vi "SemiGreedy_Filters_(Top_Level_VI)-5.vi"(5 "[IN] Max angle":dbl, 6 "[IN] Dot matrix with statuses \nfor potentially moving dots":i16[][](array[numeric]), 7 "[IN] Possibly\nMoving (X,Y)":dbl[][](array[numeric]), 8 "error IN":errorcluster, 9 "[IN] Areas particles\nPrimary Detected":dbl[][](array[numeric]), 10 "[IN] Primary \n(X,Y) Detected":dbl[][](array[numeric]), 11 "[IN] Grouped tracks":T1(array[cluster])) -> (0 "error OUT":errorcluster, 2 "[OUT] Processed Tracks":T1(array[cluster]), 3 "[OUT Tracks before Processing":T1(array[cluster]))   [LabVIEW 2013]
panel:
  out "# Iteration":i32
  out "Current\ngroup":i32
  out "# of corrections":i32
  out "[IN] Before Pro\ncessing Tracks":T1(array[cluster])
  out "[IN] Current Pro\ncessing Tracks":T2
  out "[OUT] Clusters for Re\nconstructed Tracks":T2
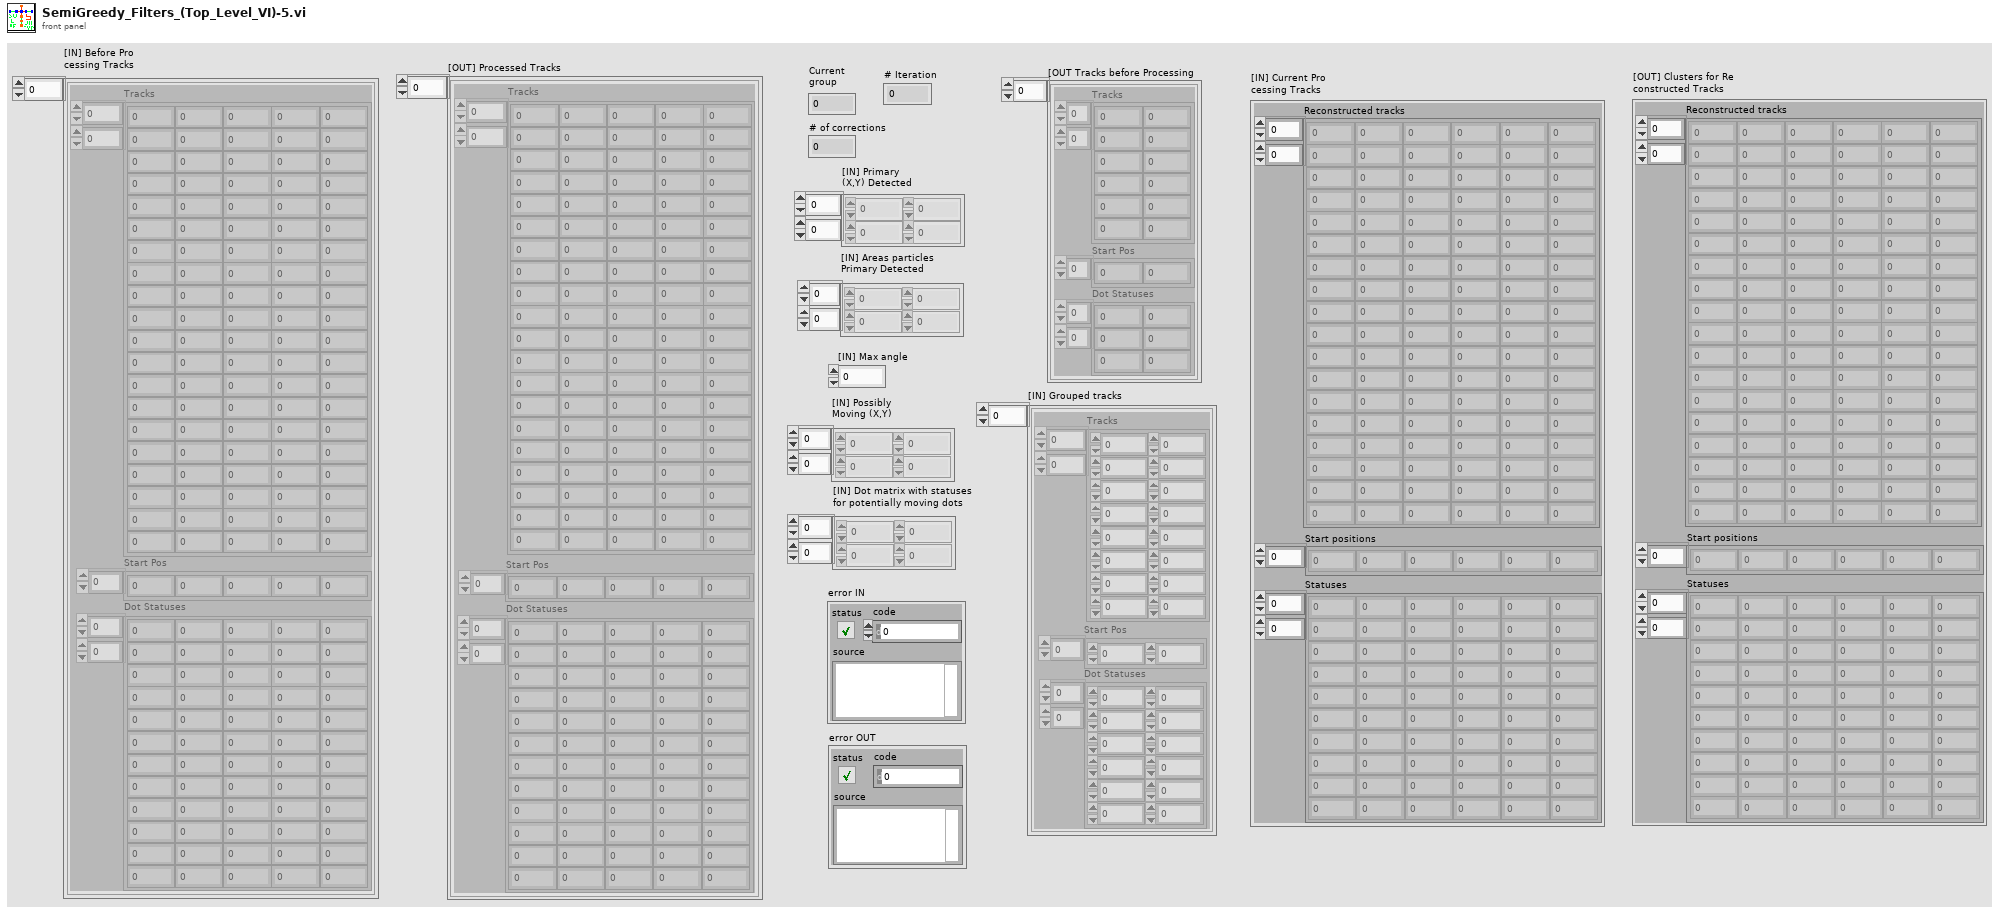
[diagram p1: front panel]
types:
  T1 = cluster{"Tracks":dbl[][], "Start Pos":i32[], "Dot Statuses":i16[][]}[]
  T2 = cluster{"Reconstructed tracks":dbl[][], "Start positions":i32[], "Statuses":i16[][]}
  T3 = cluster{"Tracks":dbl[][], "Start Pos":i32[], "Dot Statuses":i16[][]}
  T4 = cluster{"Subtrack":dbl[], "Statuses":i16[], "Start pos":i32, "Additions to cost":i32, "Track variant \nis too short":bool, "Indexes for Jumps":i32[]}[][]
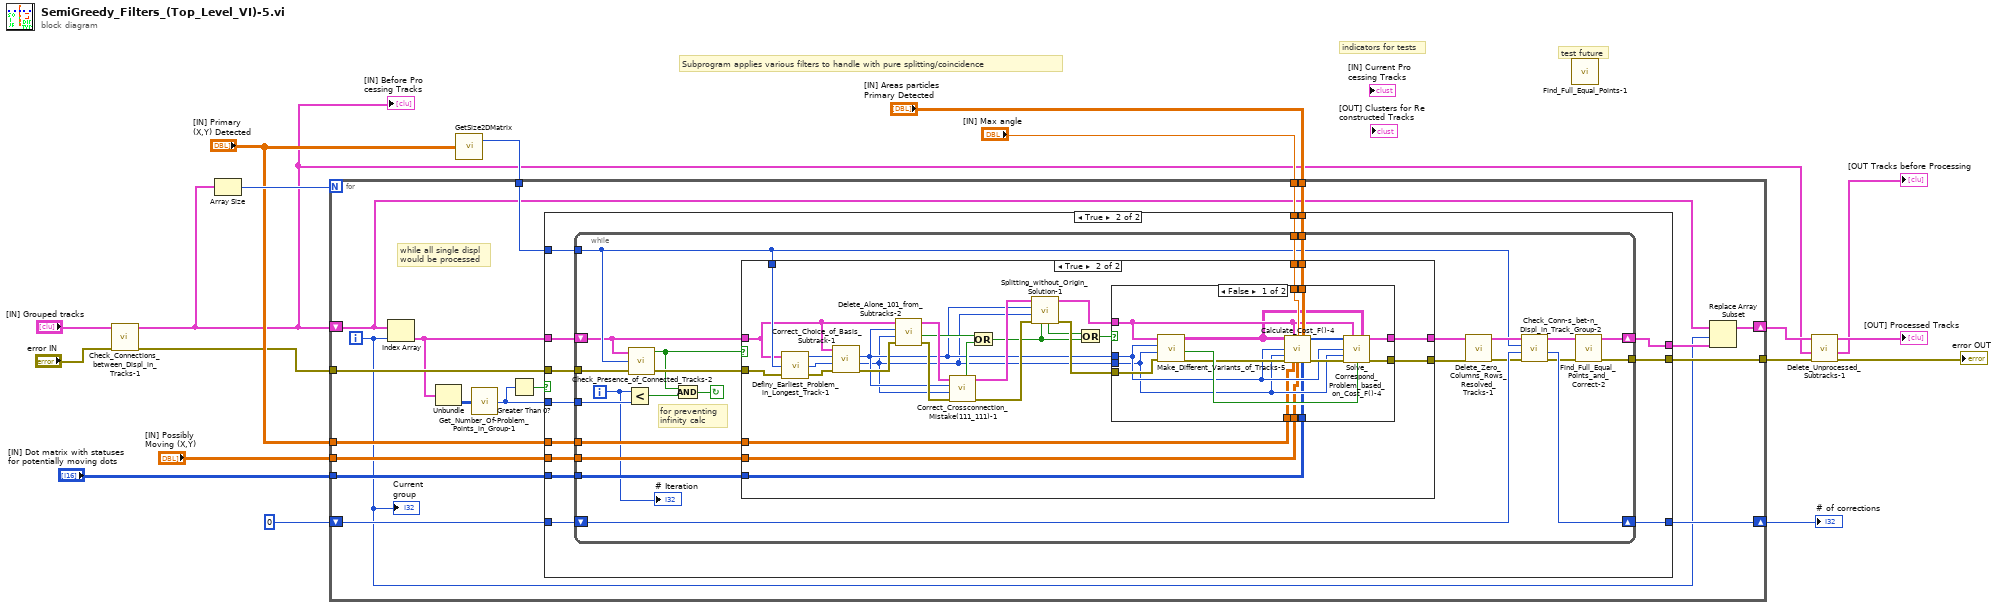
[diagram p0: block diagram]
diagram:
  # "indicators for tests"
  # "test future"
  # "Subprogram applies various filters to handle with pure splitting/coincidence"
  n1 = call "Check_Connections_between_Displ_in_Tracks-1.vi"("error IN"="error IN", "[IN] Long Connected Tracks"="[IN] Grouped tracks") -> ("error OUT"=w5:errorcluster, "[OUT] Long Connected Tracks"=w4:T1)  [unwired: 4 in]
  "[IN] Before Pro\ncessing Tracks" <- w4
  n2 = Array Size(array=w4) -> (size(s)=w18:i32)
  n3 = call "GetSize2DMatrix.vi"("Array IN (2D)"="[IN] Primary \n(X,Y) Detected") -> ("# Cols"=w10:i32)  [unwired: 1 out]
  n4 = for {
    N: w18 -> [_]
    shift-right: [w28] -> w9
    shift-left: w4 -> [w29]
    tunnel: w5 -> [w36]
    tunnel: w10 -> [w35]
    tunnel: "[IN] Areas particles\nPrimary Detected" -> [w34]
    tunnel: "[IN] Primary \n(X,Y) Detected" -> [w33]
    tunnel: "[IN] Possibly\nMoving (X,Y)" -> [w32]
    tunnel: "[IN] Dot matrix with statuses \nfor potentially moving dots" -> [w31]
    tunnel: "[IN] Max angle" -> [w30]
    tunnel: [w27] -> w8
    shift-right: [w24] -> w1
    shift-left: 0 -> [w25]
    i -> [w20]
    # "while all single displ\nwould be processed"
    n5 = Index Array(array=w29, index=w20) -> (element=w19:T3)
    n6 = Unbundle(w19) -> ("Dot Statuses"=w23:i16[][])  [unwired: 2 out]
    n7 = call "Get_Number_Of-Problem_Points_in_Group-1.vi"("[IN] Dot Statuses"=w23) -> ("[OUT] Number of problem points"=w22:i32)
    n8 = Greater Than 0?(x=w22) -> (x > 0?=w21:bool)
    n9 = case shown="True" w21 {
      tunnel: w36 -> [w38 w52]
      tunnel: w35 -> [_ w51]
      tunnel: w34 -> [_ w50]
      tunnel: w33 -> [_ w49]
      tunnel: w32 -> [_ w48]
      tunnel: w31 -> [_ w47]
      tunnel: w30 -> [_ w46]
      tunnel: [w38 w45] -> w27
      tunnel: [w39 w44] -> w26
      tunnel: w25 -> [w37 w43]
      tunnel: [w37 w42] -> w24
      tunnel: w19 -> [w39 w41]
      tunnel: w22 -> [_ w40]
      frame False {
      }
      frame True {
        n10 = while {
          tunnel: w52 -> [w59]
          tunnel: w51 -> [w56]
          tunnel: w50 -> [w76]
          tunnel: w49 -> [w75]
          tunnel: w48 -> [w74]
          tunnel: w47 -> [w73]
          tunnel: w46 -> [w72]
          shift-right: [w54] -> w44
          shift-left: w41 -> [w53]
          tunnel: [w55] -> w45
          shift-right: [w67] -> w42
          shift-left: w43 -> [w68]
          tunnel: w40 -> [w64]
          i -> [w63]
          stop <- w65 continue-if-true
          # "for preventing \ninfinity calc"
          n11 = Less?(x=w63, y=w64) -> (x < y?=w60:bool)
          n12 = call "Check_Presence_of_Connected_Tracks-2.vi"("error IN"=w59, "[IN] #of Frames"=w56, "[IN] Still connected\ntracks in group"=w53) -> ("error OUT"=w58:errorcluster, "[OUT] At least two tracks\ninside track group"=w57:bool)  [unwired: 1 in]
          n13 = And(x=w57, y=w60) -> (x .and. y?=w65:bool)
          n14 = case shown="True" w57 {
            tunnel: w58 -> [w77 w105]
            tunnel: w53 -> [w78 w93]
            tunnel: w56 -> [_ w104]
            tunnel: w76 -> [_ w99]
            tunnel: w75 -> [_ w103]
            tunnel: w74 -> [_ w102]
            tunnel: w73 -> [_ w101]
            tunnel: w72 -> [_ w100]
            tunnel: [w78 w98] -> w70
            tunnel: [w77 w97] -> w71
            frame False {
            }
            frame True {
              n15 = call "Definy_Earliest_Problem_in_Longest_Track-1.vi"("error IN"=w105, "[IN] #of Frames"=w104, "[IN] Still connected\ntracks in group"=w93) -> ("error OUT"=w94:errorcluster, "[OUT] # of Longest track\nInside the Group of Tracks"=w95:i32, "[OUT] Index of Problem\nPoint Inside Track"=w96:i32)
              n16 = call "Correct_Choice_of_Basis_Subtrack-1.vi"("error IN"=w94, "[IN] # of Longest track\nInside the Group of Tracks"=w95, "[IN] Index of Earliest \nProblem Point Inside"=w96, "[IN] Still connected\ntracks in group"=w93) -> ("error OUT"=w91:errorcluster, "[OUT] # of Correc\nted Longest Track"=w82:i32, "[OUT] # of Prob\nlem Point Inside"=w83:i32)  [unwired: 1 in]
              n17 = call "Delete_Alone_101_from_Subtracks-2.vi"("error IN"=w91, "[IN] # of Correc\nted Longest Track"=w82, "[IN] # of Prob\nlem Point Inside"=w83, "[IN] Still connected\ntracks in group"=w93) -> ("error OUT"=w90:errorcluster, "[OUT] Special case: \nAlone 101 point"=w89:bool, "[OUT] Clusters for Re\nconstructed Tracks"=w92:T2)  [unwired: 1 in]
              n18 = call "Correct_Crossconnection_Mistake(111_111)-1.vi"("error IN"=w90, "[IN] # of Track with\nFirst Problem Point"=w82, "[IN] Index of First Pro\nblem Point Inside Track"=w83, "[IN] Still connected\ntracks in group"=w92) -> ("error OUT"=w86:errorcluster, "[OUT] Clusters for Re\nconstructed Tracks"=w87:T2, "[OUT] Crossconn\nection corrected"=w88:bool)  [unwired: 5 in]
              n19 = Or(x=w89, y=w88) -> (x .or. y?=w79:bool)
              n20 = call "Splitting_without_Origin_Solution-1.vi"("[IN] Crossconn\nection corrected"=w79, "error IN"=w86, "[IN] # of Track with\nFirst Problem Point"=w82, "[IN] Index of First Pro\nblem Point Inside Track"=w83, "[IN] Still connected\ntracks in group"=w87) -> ("error OUT"=w84:errorcluster, "[OUT] Clusters for Re\nconstructed Tracks"=w85:T2, "[OUT] Problem with 11 Point\nwithout Origin Resolved"=w80:bool)  [unwired: 4 in]
              n21 = Or(x=w80, y=w79) -> (x .or. y?=w81:bool)
              n22 = case shown="False" w81 {
                tunnel: w103 -> [w108 _]
                tunnel: w102 -> [w107 _]
                tunnel: w101 -> [w106 _]
                tunnel: w100 -> [w113 _]
                tunnel: w99 -> [w114 _]
                tunnel: [w121 w123] -> w98
                tunnel: [w120 w122] -> w97
                tunnel: w83 -> [w110 _]
                tunnel: w82 -> [w109 _]
                tunnel: w84 -> [w118 w122]
                tunnel: w85 -> [w112 w123]
                frame False {
                  n23 = call "Make_Different_Variants_of_Tracks-5.vi"("error IN"=w118, "[IN] # of Longest track\nInside the Group of Tracks"=w109, "[IN] Index of Earliest \nProblem Point Inside"=w110, "[IN] Still connected\ntracks in group"=w112) -> ("error OUT"=w117:errorcluster, "[OUT] Special case!"=w119:bool, "[OUT] Subtracks"=w111:T4)  [unwired: 5 in]
                  n24 = call "Calculate_Cost_F()-4.vi"("[IN] Subtracks"=w111, "[IN] Still connected\ntracks in group"=w112, "[IN] Max angle"=w113, "[IN] Areas particles\nPrimary Detected"=w114, "[IN] Index of Earliest \nProblem Point Inside"=w110, "[IN] # of Longest track\nInside the Tracks Group"=w109, "error IN"=w117, "[IN] Primary \n(X,Y) Detected"=w108, "[IN] Potentially\nMoving (X,Y)"=w107, "[IN] Dot matrix with statuses \nfor potentially moving dots"=w106) -> ("[OUT] Cost function"=w115:i8[], "error OUT"=w116:errorcluster)  [unwired: 4 in]
                  n25 = call "Solve_Correspond_Problem_based_on_Cost_F()-4.vi"("[IN] Cost function"=w115, "[IN] Still connected\ntracks in group"=w112, "[IN] Subtracks"=w111, "[IN] Index of Earliest \nProblem Point Inside"=w110, "[IN] # of Longest track\nInside the Tracks Group"=w109, "error IN"=w116, "[IN] Special case!"=w119) -> ("[OUT] Clusters for Re\nconstructed Tracks"=w121:T2, "error OUT"=w120:errorcluster)  [unwired: 7 in]
                }
                frame True {
                }
              }
            }
          }
          n26 = call "Delete_Zero_Columns_Rows_Resolved_Tracks-1.vi"("error IN"=w71, "[IN] Clusters for Re\nconstructed Tracks"=w70) -> ("error OUT"=w66:errorcluster, "[OUT] Clusters for Re\nconstructed Tracks"=w69:T2)  [unwired: 4 in]
          n27 = call "Check_Conn-s_bet-n_Displ_in_Track_Group-2.vi"("error IN"=w66, "[IN] # of Unconne\ncted Problem points"=w68, "[IN] #of Frames"=w56, "[IN] Clusters for Re\nconstructed Tracks"=w69) -> ("error OUT"=w61:errorcluster, "[OUT] # of Unconne\ncted Problem points"=w67:i32, "[OUT] Clusters for Re\nconstructed Tracks"=w62:T2)  [unwired: 1 in]
          n28 = call "Find_Full_Equal_Points_and_Correct-2.vi"("error IN"=w61, "[IN] Clusters for Re\nconstructed Tracks"=w62) -> ("error OUT"=w55:errorcluster, "[OUT] Clusters for Re\nconstructed Tracks"=w54:T2)  [unwired: 4 in]
          "# Iteration" <- w63
        }
      }
    }
    n29 = Replace Array Subset(array=w29, new element=w26, index=w20) -> (w28:T1)
    "Current\ngroup" <- w20
  }
  "# of corrections" <- w1
  n30 = call "Find_Full_Equal_Points-1.vi"() -> ()  [unwired: 6 in, 2 out]
  n31 = call "Delete_Unprocessed_Subtracks-1.vi"("error IN"=w8, "[IN] Before Pro\ncessing Tracks"=w4, "[IN] Processed Tracks"=w9) -> ("error OUT"=→"error OUT":errorcluster, "[OUT] Before Pro\ncessing Tracks"=→"[OUT Tracks before Processing":T1, "[IN] Filtered Tracks"=→"[OUT] Processed Tracks":T1)  [unwired: 2 in]
